vi "Set Read Position.vi"(8 "error in (no error)":errorcluster, 9 "Relative? (F)":bool, 10 "Offset":i64, 11 "StringStream in":refnum<class "StringStream.lvclass">) -> (0 "error out":errorcluster, 3 "StringStream out":refnum<class "StringStream.lvclass">)   [LabVIEW 2020, in "IO.lvlib" / "StringStream.lvclass"]
uses:
  StringStream.lvclass
  StringStream.lvclass/StringStream.ctl
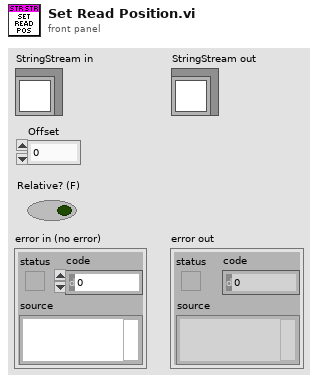
[diagram p1: front panel]
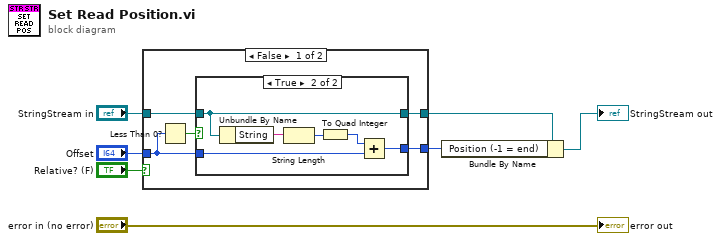
[diagram p0: block diagram]
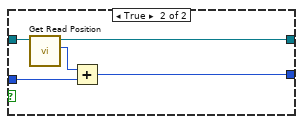
[diagram p3: hidden frame]
diagram:
  n1 = case shown="False" "Relative? (F)" {
    tunnel: "StringStream in" -> [w12 w25]
    tunnel: "Offset" -> [w10 w24]
    tunnel: [w8 w22] -> w3
    tunnel: [w9 w21] -> w2
    frame False {
      n2 = Less Than 0?(x=w10) -> (x < 0?=w11:bool)
      n3 = case shown="True" w11 {
        tunnel: w12 -> [w14 w16]
        tunnel: w10 -> [w13 w19]
        tunnel: [w13 w17] -> w9
        tunnel: [w14 w16] -> w8
        frame False {
        }
        frame True {
          n4 = Unbundle By Name(w16) -> ("String"=w20:string)
          n5 = String Length(string=w20) -> (length=w18:i32)
          n6 = To Quad Integer(1:w18) -> (0:w15:i64)
          n7 = Add(x=w15, y=w19) -> (x+y=w17:i64)
        }
      }
    }
    frame True {
      n8 = call-dynamic "Get Read Position.vi"("StringStream in"=w25) -> ("Read Position"=w23:i64, "StringStream out"=w22:refnum<class "StringStream.lvclass">)  [unwired: 8 in, 1 out]
      n9 = Add(x=w23, y=w24) -> (x+y=w21:i64)
    }
  }
  n10 = Bundle By Name(cluster=w3, "Position (-1 = end)"=w2) -> (→"StringStream out":refnum<class "StringStream.lvclass">)
  "error out" <- "error in (no error)"
